vi "time_lv2_string.vi"(1 "utc?":bool, 2 "lv_time":timestamp) -> (0 "time_string":string)   [LabVIEW 2018]
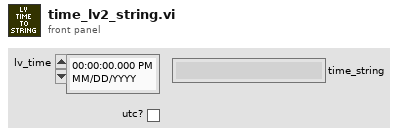
[diagram p1: front panel]
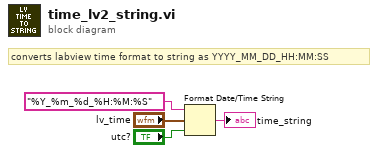
[diagram p0: block diagram]
diagram:
  # "converts labview time format to string as YYYY_MM_DD_HH:MM:SS"
  n1 = Format Date/Time String(time format string (%c)="%Y_%m_%d_%H:%M:%S", seconds (now)="lv_time", UTC format="utc?") -> (date/time string=→"time_string":string)
